vi "_Set ButtonGroupEnum Value.vi"(7 "ModeBtnRefs":refnum<vi>[](array[refnum]), 8 "error in":errorcluster, 9 "Prefix":string, 11 "Enum":variant) -> (0 "error out":errorcluster)   [LabVIEW 2017, in "ButtonGroupEnum.lvlib"]
uses:
  ButtonGroupEnum.lvlib
  _openG/_reuse_openG.lvlib
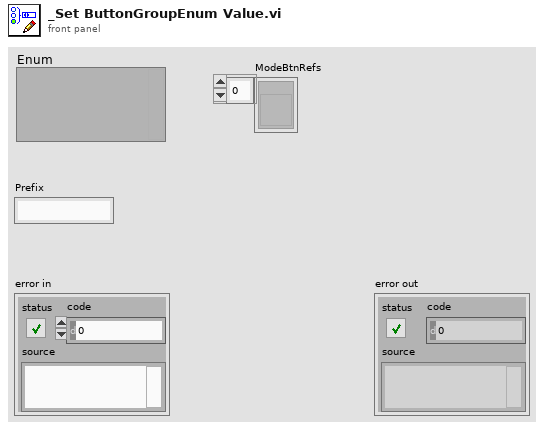
[diagram p1: front panel]
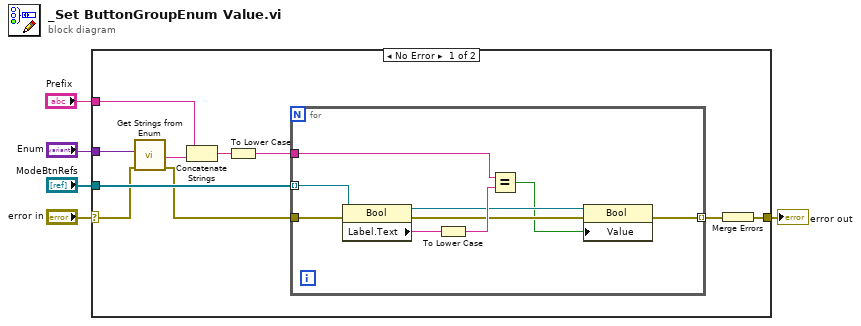
[diagram p0: block diagram]
diagram:
  n1 = case shown="No Error" "error in" {
    selector: "error in" -> [w11 w25]
    tunnel: "ModeBtnRefs" -> [w15 _]
    tunnel: [w13 w25] -> w4
    tunnel: "Enum" -> [w12 _]
    tunnel: "Prefix" -> [w8 _]
    frame No Error {
      n2 = call "Get Strings from Enum.vi"("error in (no error)"=w11, "Enum"=w12) -> ("error out"=w10:errorcluster, "String Value"=w9:string)  [unwired: 6 in, 2 out]
      n3 = Concatenate Strings(w8, w9) -> (w7:string)
      n4 = To Lower Case(string=w7) -> (all lower case string=w6:string)
      n5 = for {
        tunnel: w15 -> [w24] mode=indexing
        tunnel: [w18] -> w14 mode=indexing
        tunnel: w10 -> [w23]
        tunnel: w6 -> [w21]
        n6 = property class="Bool"(reference=w24, error in=w23) -> (reference out=w17:refnum<vi>, error out=w19:errorcluster, "Label.Text"=w22:string)
        n7 = To Lower Case(string=w22) -> (all lower case string=w20:string)
        n8 = Equal?(x=w21, y=w20) -> (x = y?=w16:bool)
        n9 = property class="Bool"(reference=w17, error in=w19, "Value"=w16) -> (error out=w18:errorcluster)  [unwired: 1 out]
      }
      n10 = Merge Errors(w14) -> (w13:errorcluster)
    }
    frame Error {
    }
  }
  "error out" <- w4
